vi "Parse String.vi"(0 "JSON String":string, 5 "Index In":i32, 11 "error in (no error)":errorcluster) -> (4 "Variant out":variant, 6 "Index Out":i32, 10 "Parsed String":string, 15 "error out":errorcluster)   [LabVIEW 2017, in "Variant JSON API.lvlib"]
uses:
  Variant JSON API.lvlib
  Errors.ctl
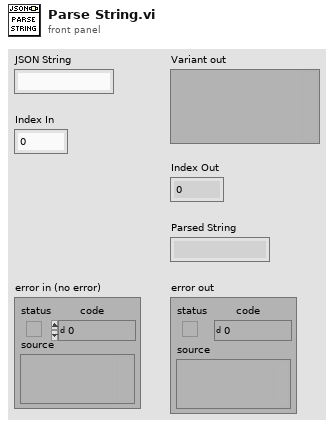
[diagram p1: front panel]
types:
  T1 = typedef "Variant JSON API.lvlib/Errors.ctl" = enum16{"No key", "Key path type", "Array OOB", "Type Mismatch", "Invalid Token", "Invalid Value"}
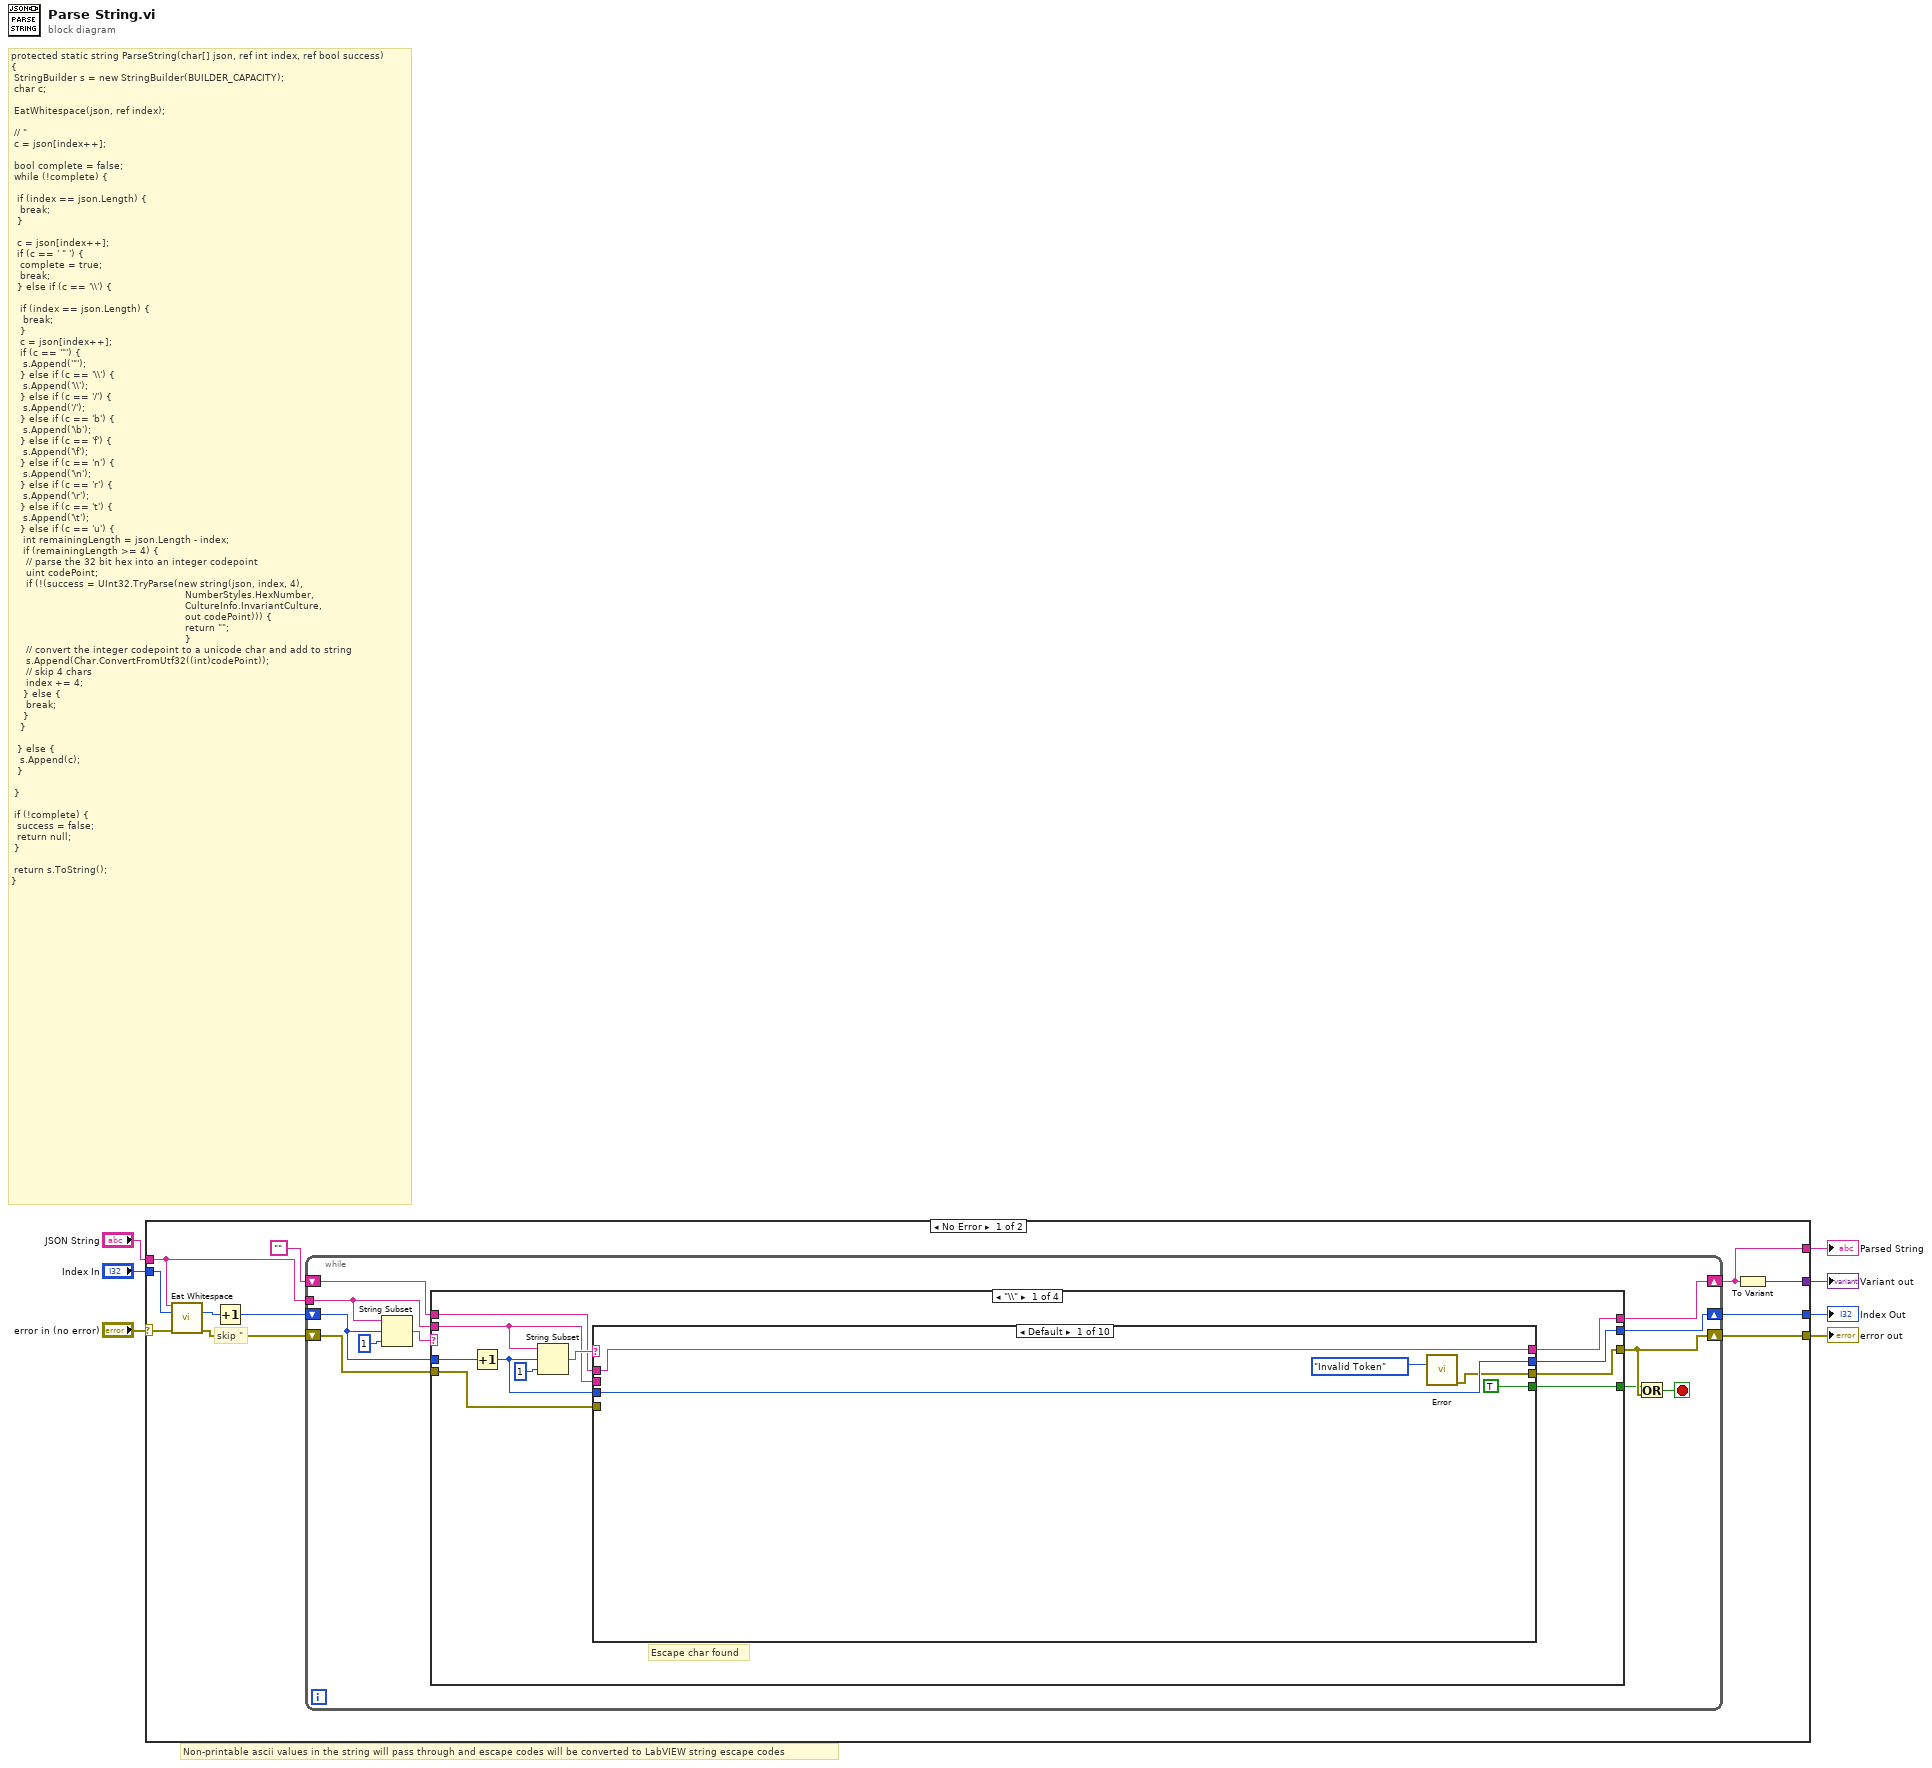
[diagram p0: block diagram]
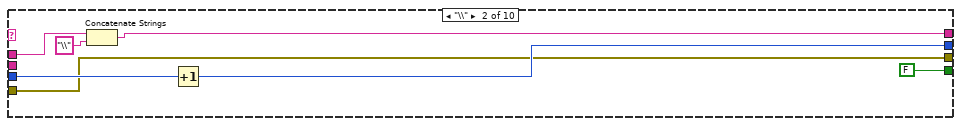
[diagram p2: hidden frame]
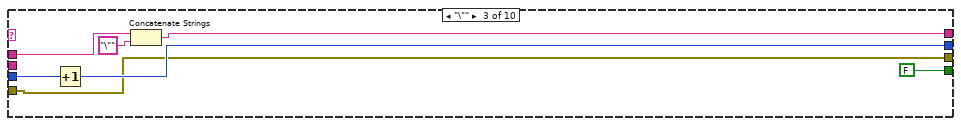
[diagram p3: hidden frame]
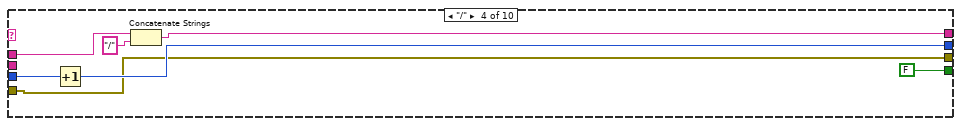
[diagram p4: hidden frame]
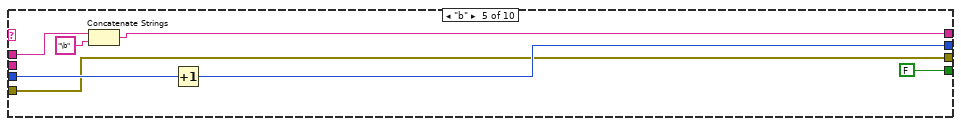
[diagram p5: hidden frame]
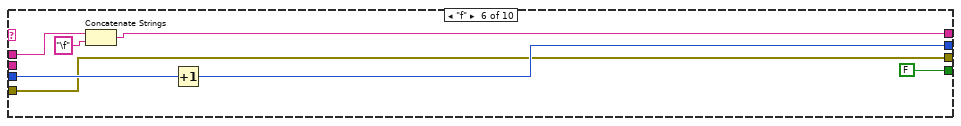
[diagram p6: hidden frame]
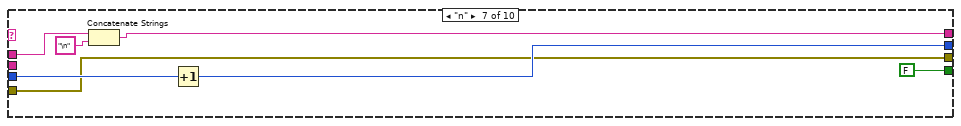
[diagram p7: hidden frame]
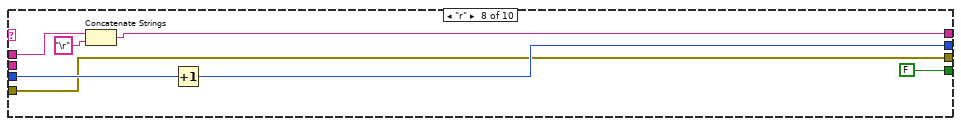
[diagram p8: hidden frame]
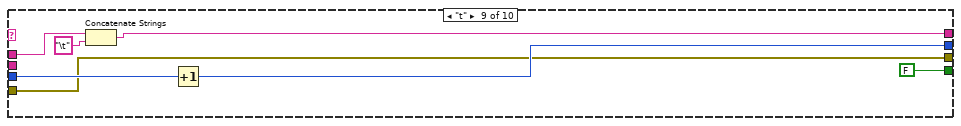
[diagram p9: hidden frame]
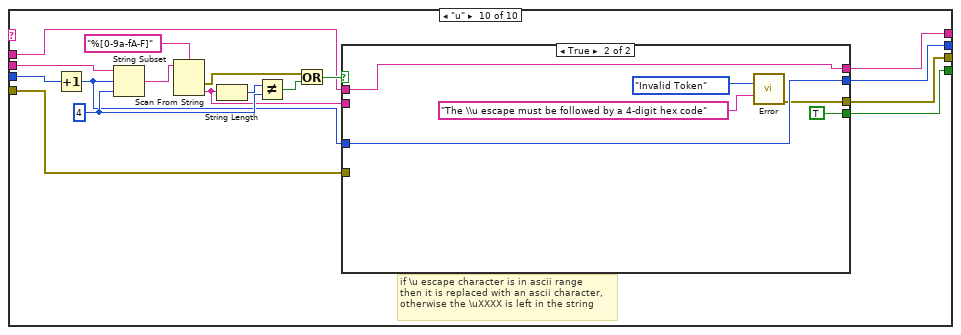
[diagram p10: hidden frame]
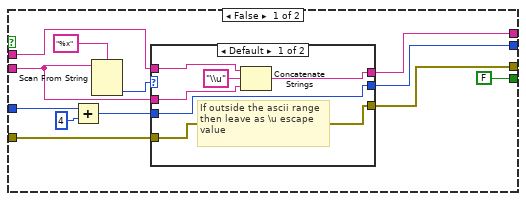
[diagram p11: hidden frame]
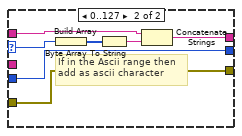
[diagram p12: hidden frame]
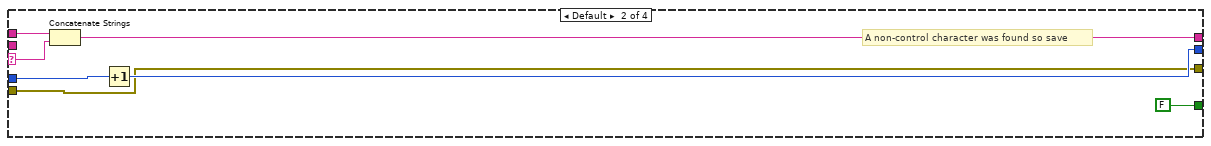
[diagram p13: hidden frame]
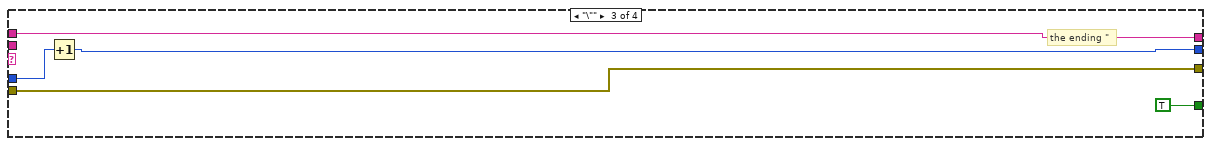
[diagram p14: hidden frame]
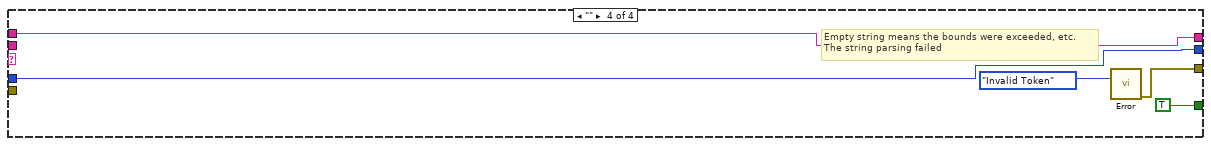
[diagram p15: hidden frame]
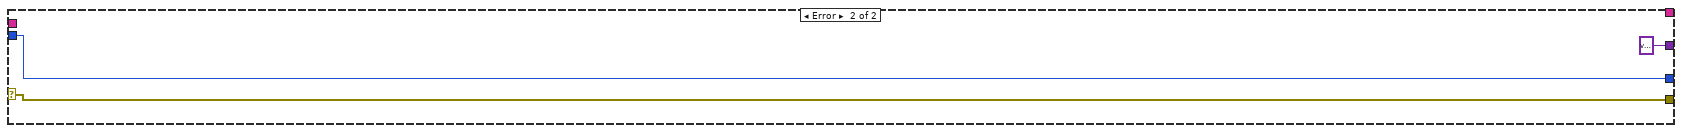
[diagram p16: hidden frame]
diagram:
  # "Non-printable ascii values in the string will pass through and escape codes will be converted to LabVIEW string escape codes"
  # "protected static string ParseString(char[] json, ref int index, ref bool success)\n{\n\tStringBuilder s = new StringBuilder(BUILDER_CAPACITY);\n\tchar c;\n\n\tEatWhitespace(json, ref index);\n\n\t// \"\n\tc = json[index++];\n\n\tbool complete = false;\n\twhile (!complete) {\n\n\t\tif (index == json.Length) {\n\t\t\tbreak;\n\t\t}\n\n\t\tc = json[index++];\n\t\tif (c == ' \" ') {\n\t\t\tcomplete = true;\n\t\t\tbreak;\n\t\t} else if (c == '\\\\') {\n\n\t\t\tif (index == json.Length) {\n\t\t\t\tbreak;\n\t\t\t}\n\t\t\tc = json[index++];\n\t\t\tif (c == '\"') {\n\t\t\t\ts.Append('\"');\n\t\t\t} else if (c == '\\\\') {\n\t\t\t\ts.Append('\\\\');\n\t\t\t} else if (c == '/') {\n\t\t\t\ts.Append('/');\n\t\t\t} else if (c == 'b') {\n\t\t\t\ts.Append('\\b');\n\t\t\t} else if (c == 'f') {\n\t\t\t\ts.Append('\\f');\n\t\t\t} else if (c == 'n') {\n\t\t\t\ts.Append('\\n');\n\t\t\t} else if (c == 'r') {\n\t\t\t\ts.Append('\\r');\n\t\t\t} else if (c == 't') {\n\t\t\t\ts.Append('\\t');\n\t\t\t} else if (c == 'u') {\n\t\t\t\tint remainingLength = json.Length - index;\n\t\t\t\tif (remainingLength >= 4) {\n\t\t\t\t\t// parse the 32 bit hex into an integer codepoint\n\t\t\t\t\tuint codePoint;\n\t\t\t\t\tif (!(success = UInt32.TryParse(new string(json, index, 4),\n                                                          NumberStyles.HexNumber,\n                                                          CultureInfo.InvariantCulture,\n                                                          out codePoint))) {\n\t\t\t\t\t\t                                                    return \"\";\n\t\t\t\t\t                                                     }\n\t\t\t\t\t// convert the integer codepoint to a unicode char and add to string\n\t\t\t\t\ts.Append(Char.ConvertFromUtf32((int)codePoint));\n\t\t\t\t\t// skip 4 chars\n\t\t\t\t\tindex += 4;\n\t\t\t\t} else {\n\t\t\t\t\tbreak;\n\t\t\t\t}\n\t\t\t}\n\n\t\t} else {\n\t\t\ts.Append(c);\n\t\t}\n\n\t}\n\n\tif (!complete) {\n\t\tsuccess = false;\n\t\treturn null;\n\t}\n\n\treturn s.ToString();\n}"
  n1 = case shown="No Error" "error in (no error)" {
    selector: "error in (no error)" -> [w18 w168]
    tunnel: [w11 w168] -> w6
    tunnel: "Index In" -> [w13 w169]
    tunnel: [w12 w169] -> w4
    tunnel: [w8 variant ("Variant")] -> w3
    tunnel: [w9 _] -> w2
    tunnel: "JSON String" -> [w10 _]
    frame No Error {
      # "skip \""
      n2 = call "Eat Whitespace.vi"("JSON String"=w10, "Index In"=w13, "error in (no error)"=w18) -> ("Index Out"=w17:i32, "error out"=w14:errorcluster)  [unwired: 10 in, 1 out]
      n3 = Increment(x=w17) -> (x+1=w16:i32)
      n4 = while {
        tunnel: w10 -> [w25]
        shift-right: [w26] -> w9
        shift-left: "" -> [w27]
        shift-right: [w22] -> w12
        shift-left: w16 -> [w23]
        shift-right: [w21] -> w11
        shift-left: w14 -> [w24]
        stop <- w19 stop-if-true
        n5 = String Subset(string=w25, offset (0)=w23, length (rest)=1 ("length (rest)")) -> (substring=w28:string)
        n6 = case shown="\"\\\\\"" w28 {
          selector: w28 -> [_ w155 _ _]
          tunnel: [w31 FALSE TRUE TRUE] -> w20
          tunnel: w27 -> [w37 w156 w160 w166]
          tunnel: [w36 w154 w160 w166] -> w26
          tunnel: w23 -> [w40 w153 w159 w164]
          tunnel: w25 -> [w30 _ _ _]
          tunnel: [w35 w152 w158 w164] -> w22
          tunnel: w24 -> [w33 w150 w157 _]
          tunnel: [w32 w150 w157 w163] -> w21
          frame "\\" {
            # "Escape char found"
            n7 = Increment(x=w40) -> (x+1=w34:i32)
            n8 = String Subset(string=w30, offset (0)=w34, length (rest)=1 ("length (rest)")) -> (substring=w38:string)
            n9 = case shown="Default" w38 {
              tunnel: w37 -> [w44 w52 w59 w66 w73 w80 w87 w94 w101 w109]
              tunnel: [w44 w51 w58 w65 w72 w79 w86 w93 w100 w105] -> w36
              tunnel: [w43 w48 w55 w62 w69 w76 w83 w90 w97 w103] -> w35
              tunnel: w34 -> [w43 w49 w56 w63 w70 w77 w84 w91 w98 w117]
              tunnel: w33 -> [_ w47 w54 w61 w68 w75 w82 w89 w96 w108]
              tunnel: [w42 w47 w54 w61 w68 w75 w82 w89 w96 w107] -> w32
              tunnel: [TRUE FALSE FALSE FALSE FALSE FALSE FALSE FALSE FALSE w106] -> w31
              tunnel: w30 -> [_ _ _ _ _ _ _ _ _ w118]
              frame Default {
                n10 = call "Error.vi"(5:Errors."Invalid Token") -> ("error out"=w42:errorcluster)  [unwired: 14 in]
              }
              frame "\\" {
                n11 = Concatenate Strings(w52, "\\" ("string")) -> (w51:string)
                n12 = Increment(x=w49) -> (x+1=w48:i32)
              }
              frame "\"" {
                n13 = Increment(x=w56) -> (x+1=w55:i32)
                n14 = Concatenate Strings(w59, "\"" ("string")) -> (w58:string)
              }
              frame "/" {
                n15 = Increment(x=w63) -> (x+1=w62:i32)
                n16 = Concatenate Strings(w66, "/" ("string")) -> (w65:string)
              }
              frame "b" {
                n17 = Concatenate Strings(w73, "\b" ("string")) -> (w72:string)
                n18 = Increment(x=w70) -> (x+1=w69:i32)
              }
              frame "f" {
                n19 = Concatenate Strings(w80, "\f" ("string")) -> (w79:string)
                n20 = Increment(x=w77) -> (x+1=w76:i32)
              }
              frame "n" {
                n21 = Concatenate Strings(w87, "\n" ("string")) -> (w86:string)
                n22 = Increment(x=w84) -> (x+1=w83:i32)
              }
              frame "r" {
                n23 = Concatenate Strings(w94, "\r" ("string")) -> (w93:string)
                n24 = Increment(x=w91) -> (x+1=w90:i32)
              }
              frame "t" {
                n25 = Concatenate Strings(w101, "\t" ("string")) -> (w100:string)
                n26 = Increment(x=w98) -> (x+1=w97:i32)
              }
              frame "u" {
                w111 = 4 ("length (rest)")
                # "if \\u escape character is in ascii range\nthen it is replaced with an ascii character,\notherwise the \\uXXXX is left in the string"
                n27 = Increment(x=w117) -> (x+1=w104:i32)
                n28 = String Subset(string=w118, offset (0)=w104, length (rest)=w111) -> (substring=w116:string)
                n29 = Scan From String(format string="%[0-9a-fA-F]", input string=w116) -> (error out=w112:errorcluster, output 1=w102:string)  [unwired: 3 in, 2 out]
                n30 = String Length(string=w102) -> (length=w114:i32)
                n31 = Not Equal?(x=w114, y=w111) -> (x != y?=w113:bool)
                n32 = Or(x=w112, y=w113) -> (x .or. y?=w110:bool)
                n33 = case shown="True" w110 {
                  tunnel: w109 -> [w127 w148]
                  tunnel: w108 -> [w125 _]
                  tunnel: [w124 w144] -> w107
                  tunnel: [FALSE TRUE] -> w106
                  tunnel: [w126 w148] -> w105
                  tunnel: w104 -> [w120 w147]
                  tunnel: [w123 w147] -> w103
                  tunnel: w102 -> [w122 _]
                  frame False {
                    n34 = Add(x=w120, y=4) -> (x+y=w119:i32)
                    n35 = Scan From String(format string="%x", input string=w122) -> (output 1=w128:u32)  [unwired: 3 in, 3 out]
                    n36 = case shown="Default" w128 {
                      selector: w128 -> [_ w143]
                      tunnel: w127 -> [w133 w141]
                      tunnel: [w134 w140] -> w126
                      tunnel: w125 -> [w135 w139]
                      tunnel: [w135 w139] -> w124
                      tunnel: [w136 w137] -> w123
                      tunnel: w122 -> [w131 _]
                      tunnel: w119 -> [w136 w137]
                      frame Default {
                        # "If outside the ascii range\nthen leave as \\u escape\nvalue"
                        n37 = Concatenate Strings(w133, "\\u" ("string"), w131) -> (w134:string)
                      }
                      frame 0..127 {
                        # "If in the Ascii range then\nadd as ascii character"
                        n38 = Build Array(w143) -> (w142:u32[])
                        n39 = Byte Array To String(unsigned byte array=w142) -> (string=w138:string)
                        n40 = Concatenate Strings(w141, w138) -> (w140:string)
                      }
                    }
                  }
                  frame True {
                    n41 = call "Error.vi"(5:Errors."Invalid Token", "Data"="The \\u escape must be followed by a 4-digit hex code" ("source")) -> ("error out"=w144:errorcluster)  [unwired: 13 in]
                  }
                }
              }
            }
          }
          frame Default {
            # "A non-control character was found so save"
            n42 = Concatenate Strings(w156, w155) -> (w154:string)
            n43 = Increment(x=w153) -> (x+1=w152:i32)
          }
          frame "\"" {
            # "the ending \""
            n44 = Increment(x=w159) -> (x+1=w158:i32)
          }
          frame "" {
            # "Empty string means the bounds were exceeded, etc.\nThe string parsing failed"
            n45 = call "Error.vi"(5:Errors."Invalid Token") -> ("error out"=w163:errorcluster)  [unwired: 14 in]
          }
        }
        n46 = Or(x=w20, y=w21) -> (x .or. y?=w19:bool)
      }
      n47 = To Variant(anything=w9) -> (Variant=w8:variant)
    }
    frame Error {
    }
  }
  "error out" <- w6
  "Index Out" <- w4
  "Variant out" <- w3
  "Parsed String" <- w2
